vi "Periodic Tasks.vi"(8 "error in":errorcluster) -> ()   [LabVIEW 2017]
doc: "This VI runs in parallel to other tasks. It can contain as many user-defined periodic loops as you need. These can carry out PID or other sorts of timed response."
uses:
  Robot Global Data.vi
  <vilib>/Rock Robotics/WPI/Solenoid/WPI_SolenoidValue.ctl
  <vilib>/Rock Robotics/WPI/Solenoid/WPI_SolenoidSetEnum.vi
panel:
  in  "negInertiaScalar":dbl=1.0
  in  "Sensitivty":dbl=1.0
  in  "WheelNonLinearity":dbl=0.65
  in  "Val_Score":dbl
  in  "Val_Segurando":dbl
  in  "Val_Expelir":dbl
  in  "Val_Coletar":dbl
  # "Intake"
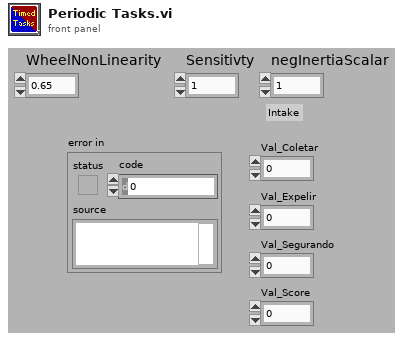
[diagram p1: front panel]
types:
  T1 = enum16{"Repouso", "Coletando", "Segurando", "Score"}
  T2 = typedef "WPI_SwitchDevRef.ctl" = cluster{"DevStatus":errorcluster, "DIO Channel":T3, "CntIndex":T4, "Normally Closed":bool}
  T3 = typedef "FPGA_DIOChannel.ctl" = enum8{"DIO 0", "DIO 1", "DIO 2", "DIO 3", "DIO 4", "DIO 5", "DIO 6", "DIO 7", "DIO 8", "DIO 9", "DIO MXP 0", "DIO MXP 1", "DIO MXP 2", "DIO MXP 3", "DIO MXP 4", "DIO MXP 5", "DIO MXP 6", "DIO MXP 7", "DIO MXP 8", "DIO MXP 9", "DIO MXP 10", "DIO MXP 11", "DIO MXP 12", "DIO MXP 13", "DIO MXP 14", "DIO MXP 15", "SPI Port CS1", "SPI Port CS2", "SPI Port CS3", "SPI Port MISO", "SPI Port MOSI", "Invalid"}
  T4 = typedef "FPGA_CounterCtrSystemIndex.ctl" = enum8{"Ctr 0", "Ctr 1", "Ctr 2", "Ctr 3", "Ctr 4", "Ctr 5", "Ctr 6", "Ctr 7", "Invalid"}
  T5 = typedef "WPI_SolenoidDevRef.ctl" = cluster{"DevStatus":errorcluster, "Pneumatics Control Module":u8, "Forward Solenoid Channel":T6, "Reverse Solenoid Channel":T6}
  T6 = typedef "WPI_SolenoidChannel.ctl" = enum8{"Solenoid 0", "Solenoid 1", "Solenoid 2", "Solenoid 3", "Solenoid 4", "Solenoid 5", "Solenoid 6", "Solenoid 7", "Invalid"}
  T7 = typedef "WPI_MotorControlDeviceRef.ctl" = cluster{"DeviceStatus":errorcluster, "Type":T8, "PWM":cluster{"PWM Channel":T9, "DeadBand":T10}, "CAN":cluster{"Device Number":u8, "SetOutput VI Ref":variant, "GetOutput VI Ref":variant, "Enable VI Ref":variant, "Disable VI Ref":variant, "Data":variant}, "Invert":bool, "DIO PWM":cluster{"PWM \"Enable\" Channel":T9, "DIOChannel":T3, "PWM Rate":dbl}}
  T8 = typedef "WPI_MotorControlType.ctl" = enum16{"PWM", "CAN", "DIO PWM"}
  T9 = typedef "FPGA_DIOPWMChannel.ctl" = enum8{"PWM 0", "PWM 1", "PWM 2", "PWM 3", "PWM 4", "PWM 5", "PWM 6", "PWM 7", "PWM 8", "PWM 9", "PWM MXP 0", "PWM MXP 1", "PWM MXP 2", "PWM MXP 3", "PWM MXP 4", "PWM MXP 5", "PWM MXP 6", "PWM MXP 7", "PWM MXP 8", "PWM MXP 9", "Invalid"}
  T10 = typedef "WPI_PWMDeadband.ctl" = cluster{"Name":string, "maxPositivePwm":i32, "minPositivePwm":i32, "centerPwm":i32, "maxNegativePwm":i32, "minNegativePwm":i32, "angularRange":u16}
  T11 = typedef "WPI_SolenoidValue.ctl" = enum16{"Off", "On", "Forward", "Reverse"}
  T12 = typedef "Button Cluster.ctl" = cluster{"Buttons[0]":bool, "Buttons[1]":bool, "Buttons[2]":bool, "Buttons[3]":bool, "Buttons[4]":bool, "Buttons[5]":bool, "Buttons[6]":bool, "Buttons[7]":bool, "Buttons[8]":bool, "Buttons[9]":bool}
  T13 = typedef "Axes Cluster.ctl" = cluster{"Axes[0]":dbl, "Axes[1]":dbl, "Axes[2]":dbl, "Axes[3]":dbl, "Axes[4]":dbl, "Axes[5]":dbl, "Axes[6]":dbl, "Axes[7]":dbl, "Axes[8]":dbl}
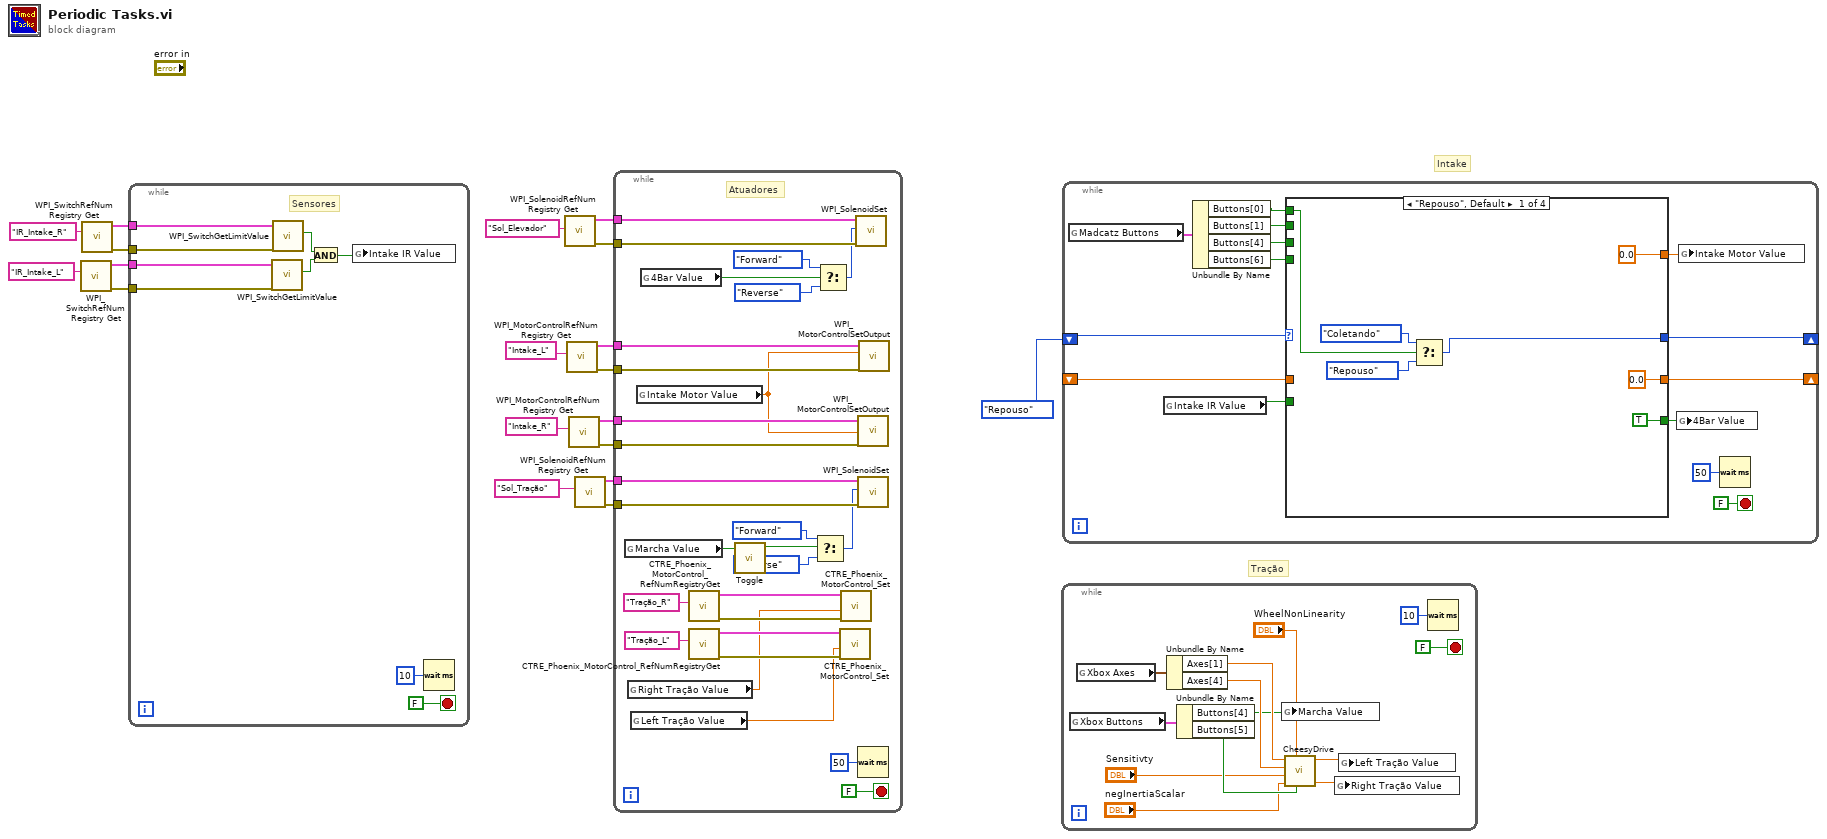
[diagram p0: block diagram]
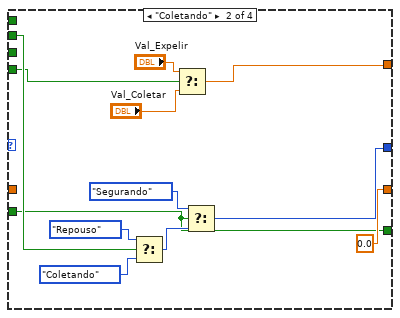
[diagram p2: hidden frame]
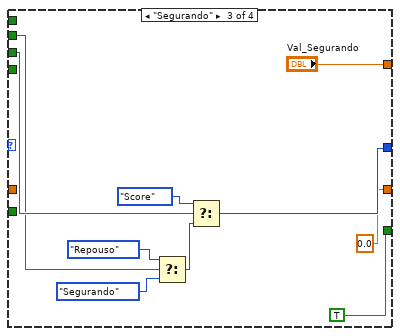
[diagram p3: hidden frame]
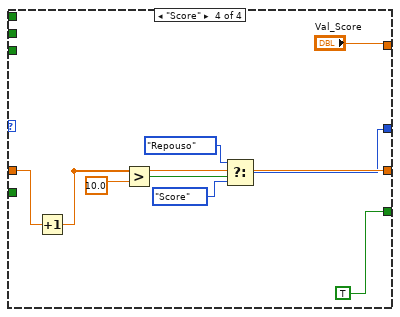
[diagram p4: hidden frame]
diagram:
  # "Tração"
  # "Intake"
  n1 = call <vilib>:"WPI_SwitchRefNum Registry Get.vi"("refnum name"="IR_Intake_L") -> ("error out"=w16:errorcluster, "SwitchDevRef"=w15:T2)  [unwired: 9 in]
  n2 = call <vilib>:"WPI_SwitchRefNum Registry Get.vi"("refnum name"="IR_Intake_R") -> ("error out"=w14:errorcluster, "SwitchDevRef"=w13:T2)  [unwired: 9 in]
  n3 = while {
    tunnel: w16 -> [w23]
    tunnel: w15 -> [w22]
    tunnel: w14 -> [w21]
    tunnel: w13 -> [w20]
    stop <- FALSE stop-if-true
    # "Sensores"
    n4 = call <vilib>:"WPI_SwitchGetLimitValue.vi"("error in (no error)"=w23, "SwitchDevRef"=w22) -> ("Switch Pressed"=w28:bool)  [unwired: 7 in, 2 out]
    n5 = call <vilib>:"WPI_SwitchGetLimitValue.vi"("error in (no error)"=w21, "SwitchDevRef"=w20) -> ("Switch Pressed"=w27:bool)  [unwired: 7 in, 2 out]
    n6 = And(x=w27, y=w28) -> (x .and. y?=w24:bool)
    n7 = global write "Robot Global Data.vi" "Intake IR Value"(w24) -> ()
    n8 = Wait (ms)(milliseconds to wait=u32 10) -> ()  [unwired: 1 out]
  }
  n9 = call <vilib>:"WPI_SolenoidRefNum Registry Get.vi"("refnum name"="Sol_Elevador") -> ("error out"=w11:errorcluster, "SolenoidDevRef"=w10:T5)  [unwired: 9 in]
  n10 = call <vilib>:"WPI_MotorControlRefNum Registry Get.vi"("refnum name"="Intake_L") -> ("error out"=w9:errorcluster, "MotorControlDevRef"=w8:T7)  [unwired: 9 in]
  n11 = call <vilib>:"WPI_MotorControlRefNum Registry Get.vi"("refnum name"="Intake_R") -> ("error out"=w4:errorcluster, "MotorControlDevRef"=w5:T7)  [unwired: 9 in]
  n12 = call <vilib>:"WPI_SolenoidRefNum Registry Get.vi"("refnum name"="Sol_Tração") -> ("error out"=w1:errorcluster, "SolenoidDevRef"=w2:T5)  [unwired: 9 in]
  n13 = while {
    tunnel: w11 -> [w56]
    tunnel: w10 -> [w55]
    tunnel: w9 -> [w50]
    tunnel: w8 -> [w49]
    tunnel: w5 -> [w48]
    tunnel: w4 -> [w47]
    tunnel: w2 -> [w41]
    tunnel: w1 -> [w40]
    stop <- FALSE stop-if-true
    # "Atuadores"
    n14 = global read "Robot Global Data.vi" "Marcha Value"() -> (w38:bool)
    n15 = global read "Robot Global Data.vi" "Right Tração Value"() -> (w30:dbl)
    n16 = global read "Robot Global Data.vi" "Left Tração Value"() -> (w29:dbl)
    n17 = global read "Robot Global Data.vi" "Intake Motor Value"() -> (w46:dbl)
    n18 = global read "Robot Global Data.vi" "4Bar Value"() -> (w51:bool)
    n19 = call <vilib>:"CTRE_Phoenix_MotorControl_RefNumRegistryGet.vi"("refnum name"="Tração_R") -> ("error out"=w31:errorcluster, "PhoenixMotorControlDevRef"=w33:T7)  [unwired: 9 in]
    n20 = call <vilib>:"CTRE_Phoenix_MotorControl_RefNumRegistryGet.vi"("refnum name"="Tração_L") -> ("error out"=w32:errorcluster, "PhoenixMotorControlDevRef"=w34:T7)  [unwired: 9 in]
    n21 = call "Toggle.vi"("In"=w38) -> ("Toggled"=w37:bool)  [unwired: 10 in]
    n22 = Select(t=WPI_SolenoidValue."Forward" ("Value"), s=w37, f=WPI_SolenoidValue."Reverse" ("Value")) -> (s? t:f=w39:T11)
    n23 = Select(t=WPI_SolenoidValue."Forward" ("Value"), s=w51, f=WPI_SolenoidValue."Reverse" ("Value")) -> (s? t:f=w54:T11)
    n24 = call <vilib>:"CTRE_Phoenix_MotorControl_Set.vi"("error in (no error)"=w32, "Output"=w29, "PhoenixMotorControlDevRef"=w34) -> ()  [unwired: 7 in, 2 out]
    n25 = call <vilib>:"CTRE_Phoenix_MotorControl_Set.vi"("error in (no error)"=w31, "Output"=w30, "PhoenixMotorControlDevRef"=w33) -> ()  [unwired: 7 in, 2 out]
    n26 = call-poly <vilib>:"WPI_SolenoidSet.vi"("error in (no error)"=w56, "Value"=w54, "SolenoidDevRef"=w55) -> ()  [unwired: 7 in, 2 out]
    n27 = call <vilib>:"WPI_MotorControlSetOutput.vi"("error in (no error)"=w47, "Output"=w46, "MotorControlDevRef"=w48) -> ()  [unwired: 6 in, 3 out]
    n28 = call-poly <vilib>:"WPI_SolenoidSet.vi"("error in (no error)"=w40, "Value"=w39, "SolenoidDevRef"=w41) -> ()  [unwired: 7 in, 2 out]
    n29 = Wait (ms)(milliseconds to wait=u32 50) -> ()  [unwired: 1 out]
    n30 = call <vilib>:"WPI_MotorControlSetOutput.vi"("error in (no error)"=w50, "Output"=w46, "MotorControlDevRef"=w49) -> ()  [unwired: 6 in, 3 out]
  }
  n31 = while {
    stop <- FALSE stop-if-true
    n32 = global read "Robot Global Data.vi" "Xbox Buttons"() -> (w65:T12)
    n33 = global read "Robot Global Data.vi" "Xbox Axes"() -> (w69:T13)
    n34 = Unbundle By Name(w69) -> ("Axes[1]"=w68:dbl, "Axes[4]"=w67:dbl)
    n35 = Unbundle By Name(w65) -> ("Buttons[4]"=w63:bool, "Buttons[5]"=w64:bool)
    n36 = global write "Robot Global Data.vi" "Marcha Value"(w63) -> ()
    n37 = call "CheesyDrive.vi"("Quickturn"=w64, "WheelNonLinearity"="WheelNonLinearity", "negInertiaScalar"="negInertiaScalar", "Sensitivty"="Sensitivty", "Wheel"=w67, "Throttle"=w68) -> ("Right PWM"=w57:dbl, "Left PWM"=w62:dbl)  [unwired: 4 in]
    n38 = global write "Robot Global Data.vi" "Right Tração Value"(w57) -> ()
    n39 = global write "Robot Global Data.vi" "Left Tração Value"(w62) -> ()
    n40 = Wait (ms)(milliseconds to wait=u32 10) -> ()  [unwired: 1 out]
  }
  n41 = while {
    shift-right: [w78] -> _
    shift-left: T1."Repouso" -> [w83]
    shift-right: [w72] -> _
    shift-left: _ -> [w73]
    stop <- FALSE stop-if-true
    n42 = global read "Robot Global Data.vi" "Madcatz Buttons"() -> (w80:T12)
    n43 = global read "Robot Global Data.vi" "Intake IR Value"() -> (w76:bool)
    n44 = Unbundle By Name(w80) -> ("Buttons[0]"=w79:bool, "Buttons[1]"=w77:bool, "Buttons[4]"=w74:bool, "Buttons[6]"=w75:bool)
    n45 = case shown="\"Repouso\", Default" w83 {
      tunnel: w79 -> [w90 _ _ _]
      tunnel: [w87 w98 w106 w115] -> w78
      tunnel: w77 -> [_ w101 w110 _]
      tunnel: w76 -> [_ w91 _ _]
      tunnel: w75 -> [_ w97 _ _]
      tunnel: w74 -> [_ _ w112 _]
      tunnel: w73 -> [_ _ _ w121]
      tunnel: [0.0 0.0 0.0 w120] -> w72
      tunnel: [0.0 w92 "Val_Segurando" "Val_Score"] -> w71
      tunnel: [TRUE w91 TRUE TRUE] -> w70
      frame "Repouso", Default {
        n46 = Select(t=T1."Coletando", s=w90, f=T1."Repouso") -> (s? t:f=w87:T1)
      }
      frame "Coletando" {
        n47 = Select(t=T1."Repouso", s=w101, f=T1."Coletando") -> (s? t:f=w94:T1)
        n48 = Select(t="Val_Expelir", s=w97, f="Val_Coletar") -> (s? t:f=w92:dbl)
        n49 = Select(t=T1."Segurando", s=w91, f=w94) -> (s? t:f=w98:T1)
      }
      frame "Segurando" {
        n50 = Select(t=T1."Repouso", s=w110, f=T1."Segurando") -> (s? t:f=w109:T1)
        n51 = Select(t=T1."Score", s=w112, f=w109) -> (s? t:f=w106:T1)
      }
      frame "Score" {
        n52 = Increment(x=w121) -> (x+1=w120:dbl)
        n53 = Greater?(x=w120, y=10.0) -> (0:w118:bool)
        n54 = Select(t=T1."Repouso", s=w118, f=T1."Score") -> (s? t:f=w115:T1)
      }
    }
    n55 = global write "Robot Global Data.vi" "4Bar Value"(w70) -> ()
    n56 = global write "Robot Global Data.vi" "Intake Motor Value"(w71) -> ()
    n57 = Wait (ms)(milliseconds to wait=u32 50) -> ()  [unwired: 1 out]
  }
